vi "Modify Speed By Step Divide (uSMC).vi"(1 "Step":u8, 2 "Speed":dbl) -> (0 "speed":dbl)   [LabVIEW 2010, in "SignalWriterMH110203USBStepperMotor.lvclass"]
uses:
  SignalWriterMH110203USBStepperMotor.lvclass
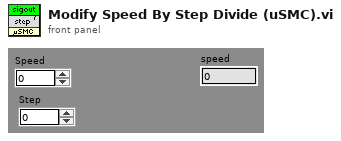
[diagram p1: front panel]
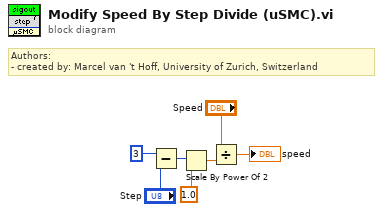
[diagram p0: block diagram]
diagram:
  # "Authors: \n- created by: Marcel van 't Hoff, University of Zurich, Switzerland"
  n1 = Subtract(x=u8 3, y="Step") -> (x-y=w4:u8)
  n2 = Scale By Power Of 2(n=w4, x=1.0) -> (x*2^n=w5:dbl)
  n3 = Divide(x="Speed", y=w5) -> (x/y=→"speed":dbl)
